vi "PointToRegisters.vi"(4 "Calibration":T2={"XHP ChirpGain"=1.0, "YHP ChirpGain"=1.0, "XLP ChirpGain"=1.0, "YLP ChirpGain"=1.0}, 5 "LP Center Frequency":u32=858993459 format="%x", 6 "Mode":enum16{"Normal", "Config"}(ring), 7 "HP Center Frequency":u32=805306367 format="%x", 8 "Range":u32 format="%x", 9 "WriteSize":enum16{"1", "2", "4"}(ring)=enum."4", 10 "UpdatesPerPoint":u32=2000, 11 "Point":cluster{"X":i32, "Y":i32, "Z":i32}) -> (0 "settings":T1 {"YLP_RR" format="%x"; "YLP_FR" format="%x"; "YHP_RR" format="%x"; "YHP_FR" format="%x"; "XLP_RR" format="%x"; "XLP_FR" format="%x"; "XHPstart" format="%x"; "XHPend" format="%x"; "XLPstart" format="%x"; "XLPend" format="%x"; "YHPstart" format="%x"; "YHPend" format="%x"; "YLPstart" format="%x"; "YLPend" format="%x"; "XHP_RR" format="%x"; "XHP_FR" format="%x"}, 1 "OutOfRange":bool, 2 "Number Registers":i16=12, 3 "Register Writes":cluster{"Address":u8, "Value":u32}[](array[cluster]))   [LabVIEW 2011]
uses:
  AODCalibration.ctl
  CoordinateSettings.ctl
panel:
  # "For 1056 AODs: 2FFFFFFF\nFor 1121 AODs: 33333333"
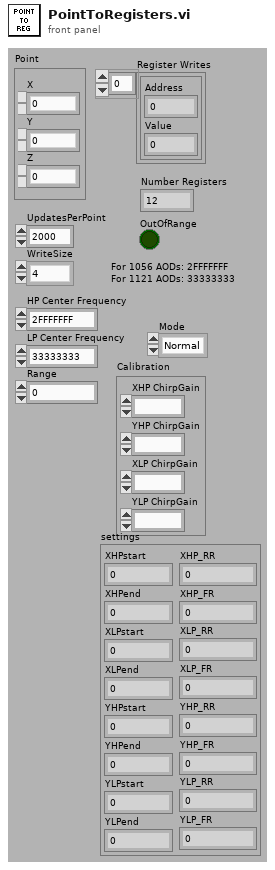
[diagram p1: front panel]
types:
  T1 = typedef "CoordinateSettings.ctl" = cluster{"XHPstart":u32, "XHPend":u32, "XLPstart":u32, "XLPend":u32, "YHPstart":u32, "YHPend":u32, "YLPstart":u32, "YLPend":u32, "XHP_RR":u32, "XHP_FR":u32, "XLP_FR":u32, "XLP_RR":u32, "YHP_FR":u32, "YHP_RR":u32, "YLP_FR":u32, "YLP_RR":u32}
  T2 = typedef "AODCalibration.ctl" = cluster{"XHP ChirpGain":fxp<+/-,16,2>, "YHP ChirpGain":fxp<+/-,16,2>, "XLP ChirpGain":fxp<+/-,16,2>, "YLP ChirpGain":fxp<+/-,16,2>}
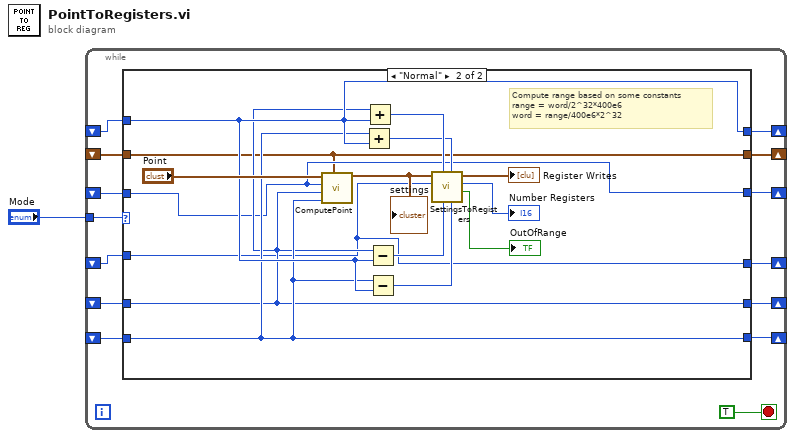
[diagram p0: block diagram]
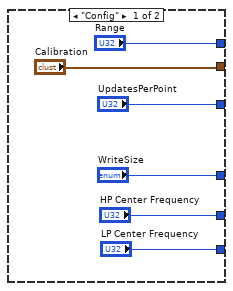
[diagram p2: hidden frame]
diagram:
  n1 = while {
    tunnel: "Mode" -> [w14]
    shift-right: [w13] -> _
    shift-left: _ -> [w9]
    shift-right: [w12] -> _
    shift-left: _ -> [w7]
    shift-right: [w11] -> _
    shift-left: _ -> [w6]
    shift-right: [w10] -> _
    shift-left: _ -> [w8]
    shift-right: [w4] -> _
    shift-left: _ -> [w5]
    shift-right: [w2] -> _
    shift-left: _ -> [w3]
    stop <- TRUE stop-if-true
    n2 = case shown="\"Normal\"" w14 {
      tunnel: ["Range" w27] -> w13
      tunnel: ["HP Center Frequency" w25] -> w12
      tunnel: ["LP Center Frequency" w26] -> w11
      tunnel: ["WriteSize" w24] -> w10
      tunnel: w9 -> [_ w27]
      tunnel: w8 -> [_ w24]
      tunnel: w7 -> [_ w25]
      tunnel: w6 -> [_ w26]
      tunnel: w5 -> [_ w23]
      tunnel: ["UpdatesPerPoint" w23] -> w4
      tunnel: w3 -> [_ w22]
      tunnel: ["Calibration" w22] -> w2
      frame "Config" {
      }
      frame "Normal" {
        # "Compute range based on some constants\nrange = word/2^32*400e6\nword = range/400e6*2^32"
        n3 = call "ComputePoint.vi"("Calibration"=w22, "LP Center Frequency"=w26, "HP Center Frequency"=w25, "UpdatesPerPoint"=w23, "Point"="Point") -> ("settings"=w35:T1)  [unwired: 6 in]
        "settings" <- w35
        n4 = Add(x=w26, y=w27) -> (x+y=w30:u32)
        n5 = Add(x=w25, y=w27) -> (x+y=w31:u32)
        n6 = Subtract(x=w25, y=w27) -> (x-y=w29:u32)
        n7 = Subtract(x=w26, y=w27) -> (x-y=w28:u32)
        n8 = call "SettingsToRegisters.vi"("LP_LowerLimit"=w28, "LP_UpperLimit"=w30, "HP_LowerLimit"=w29, "HP_UpperLimit"=w31, "WriteSize"=w24, "coordinates"=w35) -> ("OutOfRange"=→"OutOfRange":bool, "size(s)"=→"Number Registers":i32, "Register Writes"=→"Register Writes":cluster{"Address":u8, "Value":u32}[])  [unwired: 3 in]
      }
    }
  }
